vi "test Write Pin.vi"(8 "error in (no error)":errorcluster, 11 "TestCase in":refnum<class "Tester.lvclass">) -> (0 "error out":errorcluster, 3 "TestCase out":refnum<class "Tester.lvclass">)   [LabVIEW 2020, in "Tester.lvclass"]
uses:
  Tester.lvclass
  Implementations/Simulada/Simulada.lvclass
  <vilib>/addons/_JKI Toolkits/VI Tester/TestCase.llb/TestCase.lvclass
  C:/Program Files (x86)/National Instruments/LabVIEW 2020/vi.lib/addons/_JKI Toolkits/VI Tester/TestCase.llb/TestCase.lvclass
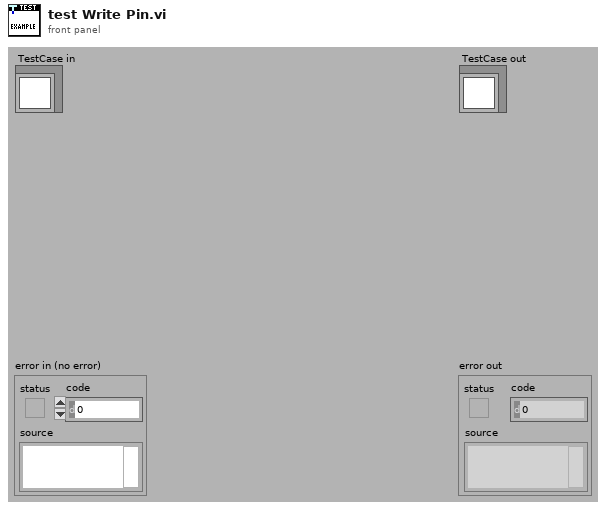
[diagram p1: front panel]
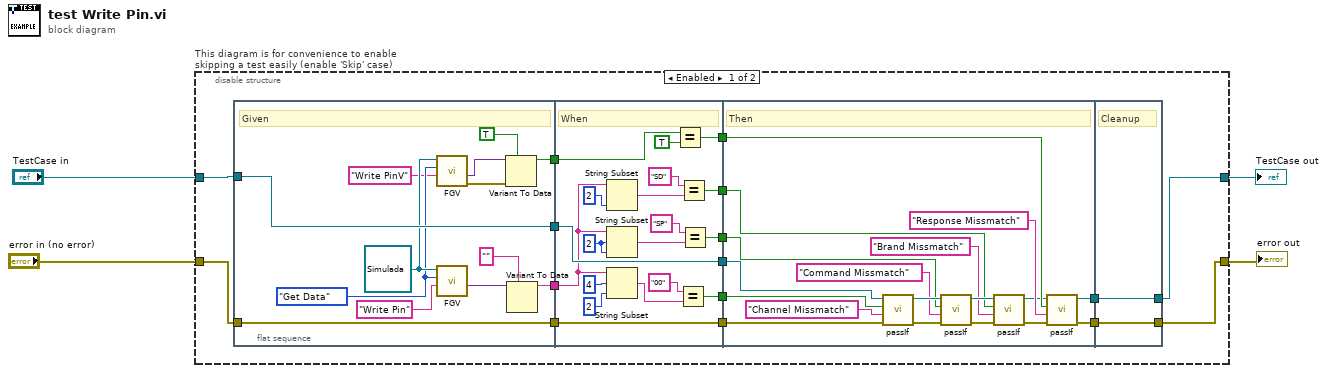
[diagram p0: block diagram]
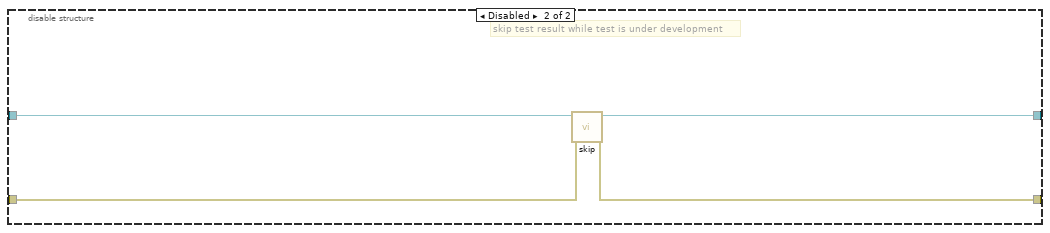
[diagram p2: hidden frame]
diagram:
  n1 = disable-structure "This diagram is for convenience to enable skipping a test easily (enable 'Skip' case)" shown="Enabled" {
    disable-tunnel: "TestCase in" -> [w8 w76]
    disable-tunnel: [w6 w74] -> w1
    disable-tunnel: [w5 w75] -> w3
    disable-tunnel: "error in (no error)" -> [w7 w73]
    frame Enabled {
      n2 = flat-sequence {
        tunnel: [w33] -> w20
        tunnel: w8 -> [w33]
        tunnel: w7 -> [w32]
        tunnel: [w32] -> w19
        tunnel: [w29] -> w18
        tunnel: [w21] -> w17
        tunnel: w20 -> [w52]
        tunnel: [w52] -> w16
        tunnel: w19 -> [w51]
        tunnel: [w51] -> w15
        tunnel: w18 -> [w47]
        tunnel: [w50] -> w14
        tunnel: [w38] -> w13
        tunnel: [w37] -> w12
        tunnel: [w36] -> w11
        tunnel: w17 -> [w35]
        tunnel: w16 -> [w66]
        tunnel: [w70] -> w10
        tunnel: w15 -> [w65]
        tunnel: [w69] -> w9
        tunnel: w14 -> [w68]
        tunnel: w13 -> [w58]
        tunnel: w12 -> [w57]
        tunnel: w11 -> [w56]
        tunnel: w10 -> [w72]
        tunnel: [w72] -> w6
        tunnel: [w71] -> w5
        tunnel: w9 -> [w71]
        frame #0 {
          w26 = enum16{"Get Data", "Set Data"}."Get Data" ("Enum")
          w27 = refnum<class "Simulada.lvclass"> refnum ("Simulada.lvclass")
          # "Given"
          n3 = call-dynamic "FGV.vi"("Simulada in"=w27, "Enum"=w26, "Name"="Write PinV") -> ("Data"=w23:variant, "error out"=w24:errorcluster)  [unwired: 5 in, 1 out]
          n4 = call-dynamic "FGV.vi"("Simulada in"=w27, "Enum"=w26, "Name"="Write Pin") -> ("Data"=w30:variant)  [unwired: 5 in, 2 out]
          n5 = Variant To Data(error in=w24, type=TRUE, Variant=w23) -> (data=w21:bool)  [unwired: 1 out]
          n6 = Variant To Data(type="", Variant=w30) -> (data=w29:string)  [unwired: 1 in, 1 out]
        }
        frame #1 {
          w40 = 2 ("length (rest)")
          # "When"
          n7 = String Subset(string=w47, length (rest)=2 ("length (rest)")) -> (substring=w46:string)  [unwired: 1 in]
          n8 = String Subset(string=w47, offset (0)=w40, length (rest)=w40) -> (substring=w45:string)
          n9 = String Subset(string=w47, offset (0)=4, length (rest)=2 ("length (rest)")) -> (substring=w44:string)
          n10 = Equal?(x=w35, y=TRUE) -> (x = y?=w50:bool)
          n11 = Equal?(x="00", y=w44) -> (x = y?=w36:bool)
          n12 = Equal?(x="SD", y=w46) -> (x = y?=w38:bool)
          n13 = Equal?(x="SP", y=w45) -> (x = y?=w37:bool)
        }
        frame #2 {
          # "Then"
          n14 = call-dynamic "passIf.vi"("error in (no error)"=w65, "message (\"\")"="Channel Missmatch" ("message (\"\")"), "pass"=w56, "TestCase in"=w66) -> ("error out"=w63:errorcluster, "TestCase out"=w64:refnum<class "Tester.lvclass">)  [unwired: 6 in]
          n15 = call-dynamic "passIf.vi"("error in (no error)"=w63, "message (\"\")"="Command Missmatch" ("message (\"\")"), "pass"=w57, "TestCase in"=w64) -> ("error out"=w61:errorcluster, "TestCase out"=w62:refnum<class "Tester.lvclass">)  [unwired: 6 in]
          n16 = call-dynamic "passIf.vi"("error in (no error)"=w61, "message (\"\")"="Brand Missmatch" ("message (\"\")"), "pass"=w58, "TestCase in"=w62) -> ("error out"=w59:errorcluster, "TestCase out"=w60:refnum<class "Tester.lvclass">)  [unwired: 6 in]
          n17 = call-dynamic "passIf.vi"("error in (no error)"=w59, "message (\"\")"="Response Missmatch" ("message (\"\")"), "pass"=w68, "TestCase in"=w60) -> ("error out"=w69:errorcluster, "TestCase out"=w70:refnum<class "Tester.lvclass">)  [unwired: 6 in]
        }
        frame #3 {
          # "Cleanup"
        }
      }
    }
    frame Disabled {
      # "skip test result while test is under development"
      n18 = call <vilib>:"skip.vi"("error in (no error)"=w73, "TestCase in"=w76) -> ("error out"=w75:errorcluster, "TestCase out"=w74:refnum<class "Tester.lvclass">)  [unwired: 8 in]
    }
  }
  "error out" <- w3
  "TestCase out" <- w1
